vi "MagCorr9225-7_FPGA.vi"(3 "dBin":fxp<+/-,36,0>, 4 "A":fxp<+,36,0>, 5 "xCORR":fxp<+,36,4>) -> (2 "rCORR":fxp<+,36,0>)   [LabVIEW 2021]
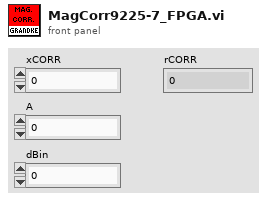
[diagram p1: front panel]
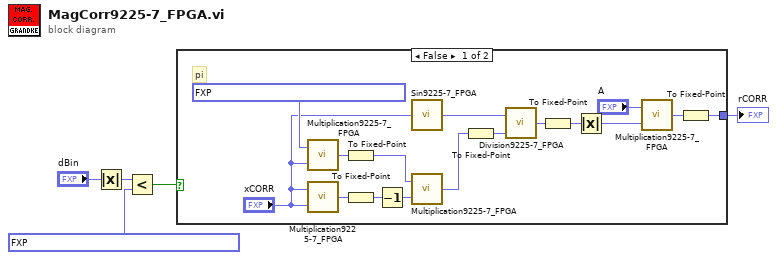
[diagram p0: block diagram]
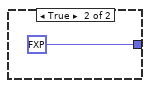
[diagram p2: hidden frame]
diagram:
  n1 = Absolute Value(x="dBin") -> (abs(x)=w4:fxp<+,36,0>)
  n2 = Less?(x=w4, y=fxp<+,36,0> 0.0010000000038417056) -> (x < y?=w3:bool)
  n3 = case shown="False" w3 {
    tunnel: [w17 fxp<+,36,0> 0.0 ("x*y")] -> w1
    frame False {
      # "pi"
      n4 = call "Multiplication9225-7_FPGA.vi"("y <+/-44,8>"="xCORR", "x <+/-47,6>"=fxp<+,36,2> 3.1415926535846666 ("x")) -> ("x*y <+/-49,13>"=w10:fxp<+/-,49,13>)
      n5 = call "Multiplication9225-7_FPGA.vi"("y <+/-44,8>"="xCORR", "x <+/-47,6>"="xCORR") -> ("x*y <+/-49,13>"=w9:fxp<+/-,49,13>)
      n6 = To Fixed-Point(number=w10) -> (fixed-point=w11:fxp<+,36,6>)  [unwired: 1 in]
      n7 = To Fixed-Point(number=w9) -> (fixed-point=w19:fxp<+,36,8>)  [unwired: 1 in]
      n8 = Decrement(x=w19) -> (x-1=w13:fxp<+,36,8>)
      n9 = call "Sin9225-7_FPGA.vi"("x [pi]"="xCORR") -> ("sin(x)"=w21:fxp<+/-,36,2>)
      n10 = call "Multiplication9225-7_FPGA.vi"("y <+/-44,8>"=w13, "x <+/-47,6>"=w11) -> ("x*y <+/-49,13>"=w12:fxp<+/-,49,13>)
      n11 = To Fixed-Point(number=w12) -> (fixed-point=w18:fxp<+,36,13>)  [unwired: 1 in]
      n12 = call "Division9225-7_FPGA.vi"("y <+/-49,13>"=w18, "x <+/-40,4>"=w21) -> ("x/y <+/-38,4>"=w20:fxp<+/-,48,14>)
      n13 = To Fixed-Point(number=w20) -> (fixed-point=w7:fxp<+/-,36,0>)  [unwired: 1 in]
      n14 = Absolute Value(x=w7) -> (abs(x)=w14:fxp<+,36,0>)
      n15 = call "Multiplication9225-7_FPGA.vi"("y <+/-44,8>"=w14, "x <+/-47,6>"="A") -> ("x*y <+/-49,13>"=w16:fxp<+/-,49,13>)
      n16 = To Fixed-Point(number=w16) -> (fixed-point=w17:fxp<+,36,0>)  [unwired: 1 in]
    }
    frame True {
    }
  }
  "rCORR" <- w1
